vi "Midpt&Orient.vi"(8 "error in (no error)":errorcluster, 9 "Enum":T1, 10 "Image In":T2, 11 "Gantry Class in":refnum<class "Gantry Class.lvclass">) -> (0 "error out":errorcluster, 1 "Midpoint":refnum<class "Vec3d Class.lvclass">, 2 "Image Out":T2, 3 "Gantry Class out":refnum<class "Gantry Class.lvclass">, 5 "Orientation":dbl)   [LabVIEW 2017, in "Gantry Class.lvclass"]
uses:
  Gantry Class.lvclass
  <vilib>/vision/Image Controls.llb/IMAQ Image.ctl
  Vec3d Class/Vec3d Class.lvclass
  Utils/Type Definitions/Object Types.ctl
  Config Manager Class/Type Definitions/Camera Enum.ctl
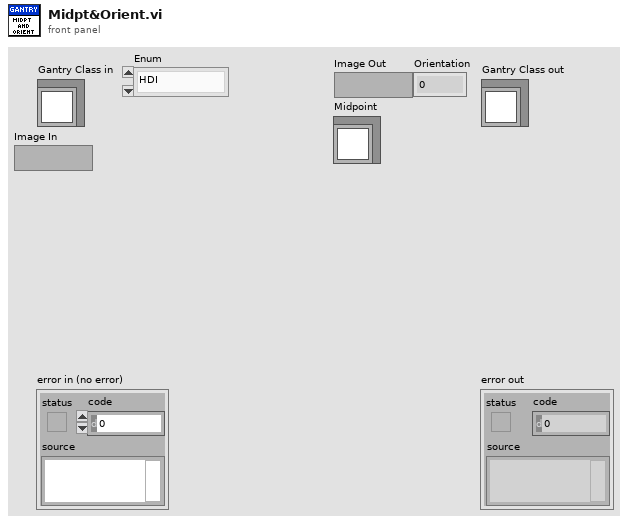
[diagram p1: front panel]
types:
  T1 = typedef "Object Types.ctl" = enum16{"HDI", "Glass Piece", "Other"}
  T2 = typedef "IMAQ Image.ctl" = refnum<image>
  T3 = typedef "Camera Enum.ctl" = enum16{"GANTRY HEAD", "NEEDLE CALIBRATION X", "NEEDLE CALIBRATION Y", "STAND CAMERA", "SIMRAN WEBCAM"}
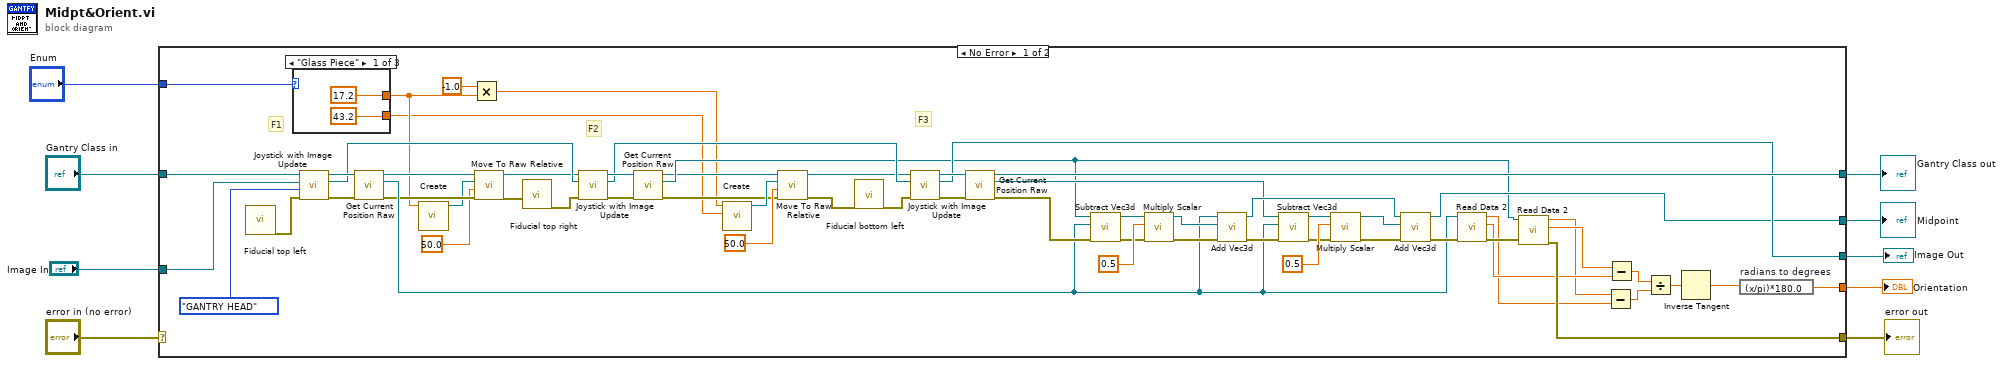
[diagram p0: block diagram]
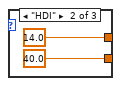
[diagram p2: hidden frame]
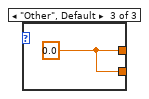
[diagram p3: hidden frame]
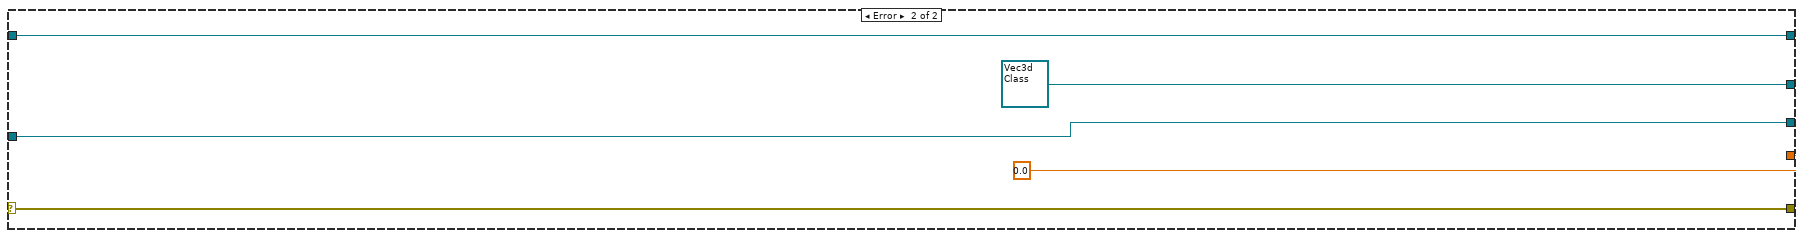
[diagram p4: hidden frame]
diagram:
  n1 = case shown="No Error" "error in (no error)" {
    selector: "error in (no error)" -> [_ w81]
    tunnel: [w34 w81] -> w8
    tunnel: "Gantry Class in" -> [w57 w80]
    tunnel: "Image In" -> [w56 w79]
    tunnel: [w36 w79] -> w5
    tunnel: [w54 w80] -> w4
    tunnel: [w35 refnum<class "Vec3d Class.lvclass"> refnum ("Vec3d Class out")] -> w3
    tunnel: [w33 0.0] -> w2
    tunnel: "Enum" -> [w26 _]
    frame No Error {
      # "F3"
      # "F2"
      # "F1"
      n2 = call "Fiducial top left"() -> ("error out"=w69:errorcluster)  [unwired: 18 in, 1 out]
      n3 = case shown="\"Glass Piece\"" w26 {
        tunnel: [17.2 ("Speed(mm/s)") 14.0 ("Speed(mm/s)") w76] -> w13
        tunnel: [43.2 ("Speed(mm/s)") 40.0 ("Speed(mm/s)") w76] -> w10
        frame "Glass Piece" {
        }
        frame "HDI" {
        }
        frame "Other", Default {
          w76 = 0.0 ("Speed(mm/s)")
        }
      }
      n4 = call-dynamic "Joystick with Image Update.vi"("error in (no error)"=w69, "Camera Name"=Camera_Enum."GANTRY HEAD", "Image In"=w56, "Gantry Class in"=w57) -> ("error out"=w70:errorcluster, "Image Out"=w59:T2, "Gantry Class out"=w71:refnum<class "Gantry Class.lvclass">)  [unwired: 5 in]
      n5 = call-dynamic "Get Current Position Raw.vi"("error in"=w70, "Gantry in"=w71) -> ("error out"=w24:errorcluster, "Vec3d Class out"=w31:refnum<class "Vec3d Class.lvclass">, "Gantry out"=w25:refnum<class "Gantry Class.lvclass">)  [unwired: 7 in]
      n6 = call "Create.vi"("X"=w13) -> ("Vec3d Class out"=w20:refnum<class "Vec3d Class.lvclass">)  [unwired: 9 in, 1 out]
      n7 = Multiply(x=-1.0, y=w13) -> (x*y=w11:dbl)
      n8 = call-dynamic "Move To Raw Relative.vi"("error in"=w24, "Speed(mm/s)"=50.0, "Delta"=w20, "Gantry in"=w25) -> ("error out"=w23:errorcluster, "Gantry out"=w22:refnum<class "Gantry Class.lvclass">)  [unwired: 6 in]
      n9 = call "Fiducial top right"("error in (no error)"=w23) -> ("error out"=w66:errorcluster)  [unwired: 17 in, 1 out]
      n10 = call-dynamic "Joystick with Image Update.vi"("error in (no error)"=w66, "Image In"=w59, "Gantry Class in"=w22) -> ("error out"=w67:errorcluster, "Image Out"=w58:T2, "Gantry Class out"=w68:refnum<class "Gantry Class.lvclass">)  [unwired: 6 in]
      n11 = call-dynamic "Get Current Position Raw.vi"("error in"=w67, "Gantry in"=w68) -> ("error out"=w16:errorcluster, "Vec3d Class out"=w32:refnum<class "Vec3d Class.lvclass">, "Gantry out"=w17:refnum<class "Gantry Class.lvclass">)  [unwired: 7 in]
      n12 = call "Create.vi"("Y"=w10, "X"=w11) -> ("Vec3d Class out"=w18:refnum<class "Vec3d Class.lvclass">)  [unwired: 8 in, 1 out]
      n13 = call-dynamic "Move To Raw Relative.vi"("error in"=w16, "Speed(mm/s)"=50.0, "Delta"=w18, "Gantry in"=w17) -> ("error out"=w15:errorcluster, "Gantry out"=w14:refnum<class "Gantry Class.lvclass">)  [unwired: 6 in]
      n14 = call "Fiducial bottom left"("error in (no error)"=w15) -> ("error out"=w63:errorcluster)  [unwired: 17 in, 1 out]
      n15 = call-dynamic "Joystick with Image Update.vi"("error in (no error)"=w63, "Image In"=w58, "Gantry Class in"=w14) -> ("error out"=w64:errorcluster, "Image Out"=w36:T2, "Gantry Class out"=w65:refnum<class "Gantry Class.lvclass">)  [unwired: 6 in]
      n16 = call-dynamic "Get Current Position Raw.vi"("error in"=w64, "Gantry in"=w65) -> ("error out"=w60:errorcluster, "Vec3d Class out"=w42:refnum<class "Vec3d Class.lvclass">, "Gantry out"=w54:refnum<class "Gantry Class.lvclass">)  [unwired: 7 in]
      n17 = call "Subtract Vec3d.vi"("error in (no error)"=w60, "Vec3d in 2"=w31, "Vec3d in 1"=w32) -> ("error out"=w61:errorcluster, "Vec3d Class out"=w53:refnum<class "Vec3d Class.lvclass">)  [unwired: 7 in]
      n18 = call-dynamic "Multiply Scalar.vi"("error in"=w61, "Scale"=0.5, "Vec3d in"=w53) -> ("error out"=w52:errorcluster, "Vec3d out"=w44:refnum<class "Vec3d Class.lvclass">)  [unwired: 7 in]
      n19 = call-dynamic "Add Vec3d.vi"("error in (no error)"=w52, 10:"Vec3d Class in"=w44, 11:"Vec3d Class in"=w31) -> ("error out"=w45:errorcluster, "Vec3d Class out"=w46:refnum<class "Vec3d Class.lvclass">)  [unwired: 7 in]
      n20 = call "Subtract Vec3d.vi"("error in (no error)"=w45, "Vec3d in 2"=w31, "Vec3d in 1"=w42) -> ("error out"=w50:errorcluster, "Vec3d Class out"=w49:refnum<class "Vec3d Class.lvclass">)  [unwired: 7 in]
      n21 = call-dynamic "Multiply Scalar.vi"("error in"=w50, "Scale"=0.5, "Vec3d in"=w49) -> ("error out"=w47:errorcluster, "Vec3d out"=w48:refnum<class "Vec3d Class.lvclass">)  [unwired: 7 in]
      n22 = call-dynamic "Add Vec3d.vi"("error in (no error)"=w47, 10:"Vec3d Class in"=w48, 11:"Vec3d Class in"=w46) -> ("error out"=w43:errorcluster, "Vec3d Class out"=w35:refnum<class "Vec3d Class.lvclass">)  [unwired: 7 in]
      n23 = call-dynamic "Read Data 2.vi"("error in"=w43, "Vec3d in"=w31) -> ("error out"=w41:errorcluster, "Y"=w29:dbl, "X"=w27:dbl)  [unwired: 6 in, 1 out]
      n24 = call-dynamic "Read Data 2.vi"("error in"=w41, "Vec3d in"=w32) -> ("error out"=w34:errorcluster, "Y"=w30:dbl, "X"=w28:dbl)  [unwired: 6 in, 1 out]
      n25 = Subtract(x=w28, y=w27) -> (x-y=w39:dbl)
      n26 = Subtract(x=w30, y=w29) -> (x-y=w40:dbl)
      n27 = Divide(x=w40, y=w39) -> (x/y=w38:dbl)
      n28 = Inverse Tangent(1:w38) -> (0:w37:dbl)
      n29 = expression code="(x/pi)*180.0" "radians to degrees"(w37) -> (w33:dbl)
    }
    frame Error {
    }
  }
  "error out" <- w8
  "Gantry Class out" <- w4
  "Image Out" <- w5
  "Midpoint" <- w3
  "Orientation" <- w2
